vi "Set Display Elements.vi"(8 "Error In":errorcluster, 10 "Display Elements":refnum<class "Display Element.lvclass">[](array[class]), 11 "Display In":refnum<class "Display.lvclass">) -> (0 "Error Out":errorcluster, 3 "Display Out":refnum<class "Display.lvclass">)   [LabVIEW 2019, in "Display.lvclass"]
uses:
  Display.lvclass
  Display Element/Display Element.lvclass
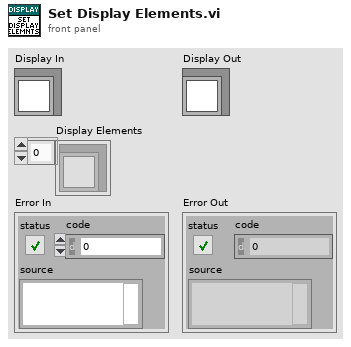
[diagram p1: front panel]
types:
  T1 = typedef "Display.lvclass/Data.ctl" = cluster{"Size":T2, "Display Elements":refnum<class "Display Element.lvclass">[], "Frame":T3}
  T2 = typedef "Display.lvclass/Size.ctl" = cluster{"Width":dbl, "Length":dbl}
  T3 = typedef "Display.lvclass/Frame.ctl" = cluster{"Matrix":u32[][]}
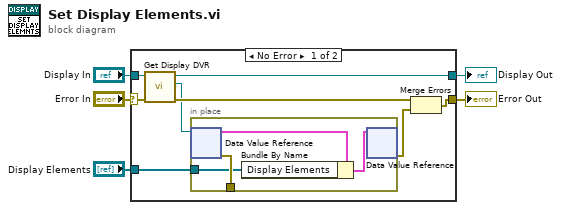
[diagram p0: block diagram]
diagram:
  n1 = case shown="No Error" "Error In" {
    selector: "Error In" -> [w10 w18]
    tunnel: [w12 w18] -> w1
    tunnel: [w7 w19] -> w2
    tunnel: "Display In" -> [w9 w19]
    tunnel: "Display Elements" -> [w11 _]
    frame No Error {
      n2 = call "Get Display DVR.vi"("Error In"=w10, "Display In"=w9) -> ("Error Out"=w8:errorcluster, "DVR"=w6:refnum<data-value>, "Display Out"=w7:refnum<class "Display.lvclass">)  [unwired: 7 in]
      n3 = in-place {
        in-place-border: [w17] -> _
        in-place-border: w11 -> [w14]
        n4 = in-place-dvr #1(w6) -> (w16:T1, w17:errorcluster)
        n5 = Bundle By Name(cluster=w16, "Display Elements"=w14) -> (w15:T1)
        n6 = in-place-dvr #1(w15) -> (w13:errorcluster)  [unwired: 1 out]
      }
      n7 = Merge Errors(w8, w13) -> (w12:errorcluster)
    }
    frame Error {
    }
  }
  "Display Out" <- w2
  "Error Out" <- w1
